vi "GetTodaysDate.vi"() -> (0 "time string":string, 3 "concatenated string":string)   [LabVIEW 2018, in "RW_Protocols.lvlib"]
uses:
  RW_Protocols.lvlib
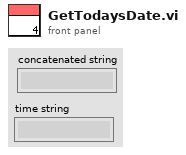
[diagram p1: front panel]
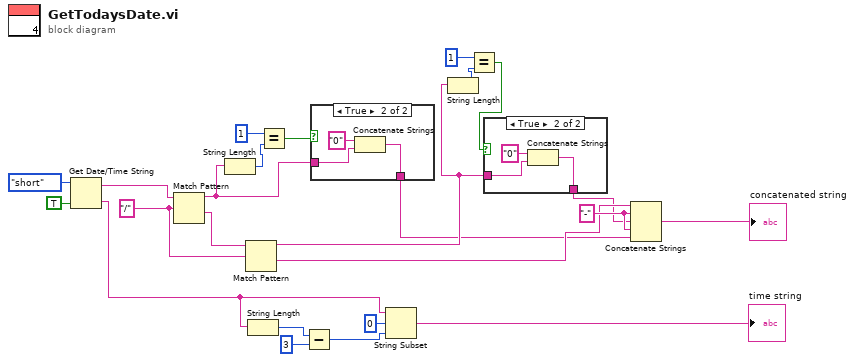
[diagram p0: block diagram]
diagram:
  w20 = "-" ("string")
  w21 = "/" ("regular expression")
  n1 = Get Date/Time String(date format (0)=enum16{"short", "long", "abbreviated"}."short", want seconds? (F)=TRUE) -> (date string=w23:string, time string=w4:string)  [unwired: 1 in]
  n2 = Match Pattern(string=w23, regular expression=w21) -> (before substring=w14:string, after substring=w22:string)  [unwired: 1 in, 2 out]
  n3 = String Length(string=w14) -> (length=w17:i32)
  n4 = Match Pattern(string=w22, regular expression=w21) -> (before substring=w13:string, after substring=w19:string)  [unwired: 1 in, 2 out]
  n5 = String Length(string=w4) -> (length=w7:i32)
  n6 = Equal?(x=1, y=w17) -> (x = y?=w15:bool)
  n7 = Subtract(x=w7, y=3) -> (x-y=w5:i32)
  n8 = case shown="True" w15 {
    tunnel: w14 -> [w25 w27]
    tunnel: [w25 w26] -> w2
    frame False {
    }
    frame True {
      n9 = Concatenate Strings("0" ("string"), w27) -> (w26:string)
    }
  }
  n10 = String Subset(string=w4, offset (0)=0, length (rest)=w5) -> (substring=→"time string":string)
  n11 = String Length(string=w13) -> (length=w11:i32)
  n12 = Equal?(x=1, y=w11) -> (x = y?=w10:bool)
  n13 = case shown="True" w10 {
    tunnel: w13 -> [w29 w31]
    tunnel: [w29 w30] -> w1
    frame False {
    }
    frame True {
      n14 = Concatenate Strings("0" ("string"), w31) -> (w30:string)
    }
  }
  n15 = Concatenate Strings(w19, w20, w1, w20, w2) -> (→"concatenated string":string)
